vi "CoolLED_by_Functions.vi"(8 "error in (no error)":errorcluster, 9 "Function":enum16{"Initialize", "Send", "Store", "Close"}(ring)) -> (0 "error out":errorcluster)   [LabVIEW 2025]
panel:
  out "Presets":bool
  out "Settings":bool
  out "Store":bool
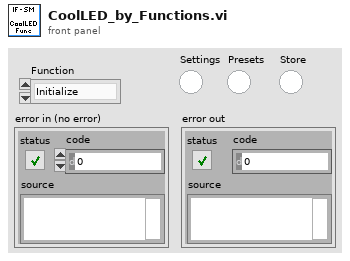
[diagram p1: front panel]
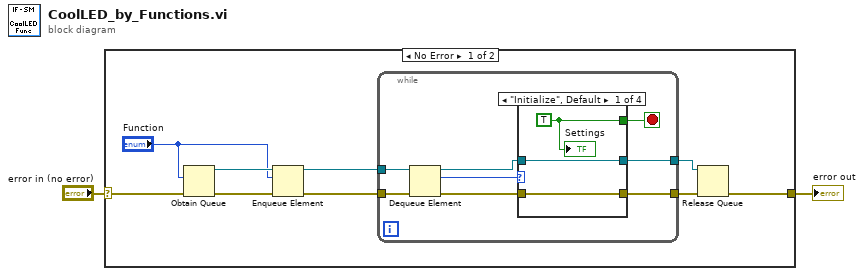
[diagram p0: block diagram]
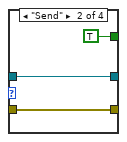
[diagram p2: hidden frame]
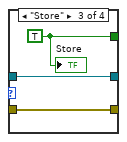
[diagram p3: hidden frame]
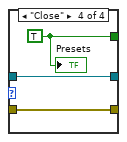
[diagram p4: hidden frame]
diagram:
  n1 = case shown="No Error" "error in (no error)" {
    selector: "error in (no error)" -> [w3 w32]
    tunnel: [w4 w32] -> w2
    frame No Error {
      n2 = Obtain Queue(element data type="Function", error in (no error)=w3) -> (queue out=w10:refnum<queue>, error out=w11:errorcluster)  [unwired: 3 in, 1 out]
      n3 = Enqueue Element(queue=w10, element="Function", error in (no error)=w11) -> (queue out=w7:refnum<queue>, error out=w9:errorcluster)  [unwired: 1 in, 1 out]
      n4 = while {
        tunnel: w9 -> [w17]
        tunnel: w7 -> [w19]
        tunnel: [w14] -> w6
        tunnel: [w13] -> w5
        stop <- w12 stop-if-true
        n5 = Dequeue Element(queue=w19, error in (no error)=w17) -> (queue out=w18:refnum<queue>, element=w15:enum16{"Initialize", "Send", "Store", "Close"}, error out=w16:errorcluster)  [unwired: 1 in, 1 out]
        n6 = case shown="\"Initialize\", Default" w15 {
          tunnel: w18 -> [w22 w25 w28 w31]
          tunnel: w16 -> [w21 w24 w27 w30]
          tunnel: [w22 w25 w28 w31] -> w14
          tunnel: [w21 w24 w27 w30] -> w13
          tunnel: [w20 TRUE w26 w29] -> w12
          frame "Initialize", Default {
            w20 = TRUE
            "Settings" <- w20
          }
          frame "Send" {
          }
          frame "Store" {
            w26 = TRUE
            "Store" <- w26
          }
          frame "Close" {
            w29 = TRUE
            "Presets" <- w29
          }
        }
      }
      n7 = Release Queue(queue=w6, error in (no error)=w5) -> (error out=w4:errorcluster)  [unwired: 1 in, 2 out]
    }
    frame Error {
    }
  }
  "error out" <- w2
